vi "CalculateHaversineDistance.vi"(10 "Target Waypoint":cluster{"Longitude":dbl, "Latitude":dbl} {"Latitude" format="%#_8g"}, 11 "Robot Position":cluster{"Longitude":dbl, "Latitude":dbl}) -> (3 "distance (dm)":dbl)   [LabVIEW 2011]
panel:
  out "Robot Latitude":dbl
  out "Robot Longitude":dbl
  out "Target Latitude":dbl
  out "Target Longitude":dbl
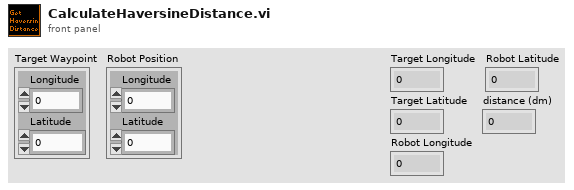
[diagram p1: front panel]
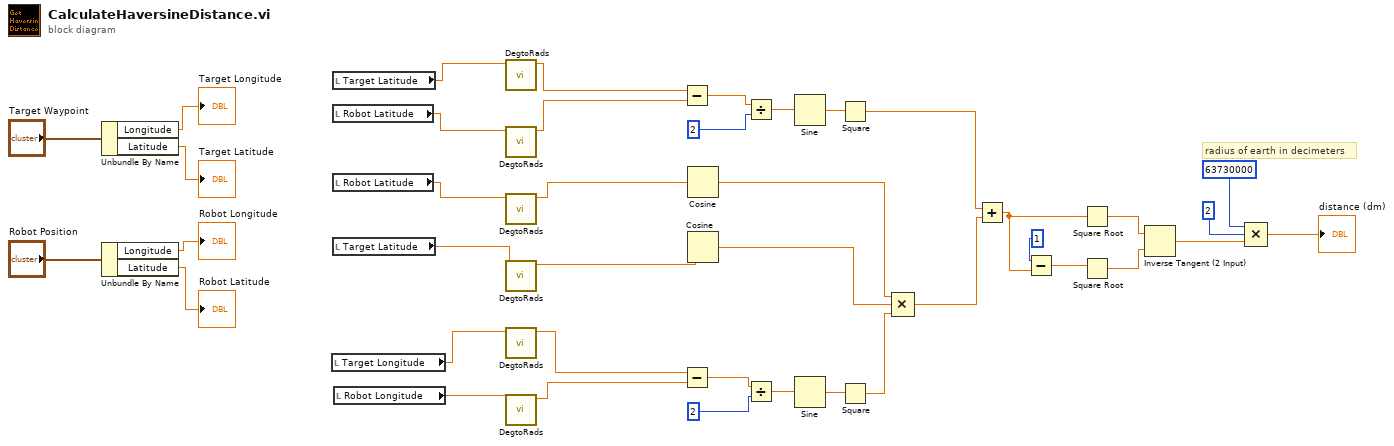
[diagram p0: block diagram]
diagram:
  # "radius of earth in decimeters"
  n1 = Unbundle By Name("Target Waypoint") -> ("Longitude"=→"Target Longitude":dbl, "Latitude"=→"Target Latitude":dbl)
  n2 = Unbundle By Name("Robot Position") -> ("Longitude"=→"Robot Longitude":dbl, "Latitude"=→"Robot Latitude":dbl)
  n3 = local read "Target Longitude"() -> (w4:dbl)
  n4 = local read "Target Latitude"() -> (w12:dbl)
  n5 = local read "Robot Latitude"() -> (w10:dbl)
  n6 = local read "Robot Latitude"() -> (w8:dbl)
  n7 = local read "Target Latitude"() -> (w6:dbl)
  n8 = local read "Robot Longitude"() -> (w2:dbl)
  n9 = call "DegtoRads.vi"("Degrees in"=w12) -> ("Rads Out"=w11:dbl)  [unwired: 10 in]
  n10 = call "DegtoRads.vi"("Degrees in"=w10) -> ("Rads Out"=w9:dbl)  [unwired: 10 in]
  n11 = call "DegtoRads.vi"("Degrees in"=w8) -> ("Rads Out"=w7:dbl)  [unwired: 10 in]
  n12 = call "DegtoRads.vi"("Degrees in"=w6) -> ("Rads Out"=w5:dbl)  [unwired: 10 in]
  n13 = call "DegtoRads.vi"("Degrees in"=w4) -> ("Rads Out"=w3:dbl)  [unwired: 10 in]
  n14 = call "DegtoRads.vi"("Degrees in"=w2) -> ("Rads Out"=w1:dbl)  [unwired: 10 in]
  n15 = Subtract(x=w11, y=w9) -> (x-y=w33:dbl)
  n16 = Subtract(x=w3, y=w1) -> (x-y=w29:dbl)
  n17 = Cosine(x=w7) -> (cos(x)=w24:dbl)
  n18 = Cosine(x=w5) -> (cos(x)=w25:dbl)
  n19 = Divide(x=w33, y=2) -> (x/y=w32:dbl)
  n20 = Divide(x=w29, y=2) -> (x/y=w28:dbl)
  n21 = Sine(x=w32) -> (sin(x)=w31:dbl)
  n22 = Sine(x=w28) -> (sin(x)=w27:dbl)
  n23 = Square(x=w31) -> (x^2=w22:dbl)
  n24 = Square(x=w27) -> (x^2=w26:dbl)
  n25 = Compound Arithmetic op=MULTIPLY(w24, w25, w26) -> (w23:dbl)
  n26 = Add(x=w22, y=w23) -> (x+y=w17:dbl)
  n27 = Subtract(x=1, y=w17) -> (x-y=w16:dbl)
  n28 = Square Root(x=w17) -> (sqrt(x)=w14:dbl)
  n29 = Square Root(x=w16) -> (sqrt(x)=w13:dbl)
  n30 = Inverse Tangent (2 Input)(1:w13, 2:w14) -> (0:w15:dbl)
  n31 = Compound Arithmetic op=MULTIPLY(63730000, 2, w15) -> (→"distance (dm)":dbl)
